vi "test_eet.vi"() -> ()   [LabVIEW 2023]
panel:
  out "lrv":sgl[](array[numeric])
  out "right_ray":sgl[](array[numeric])
  out "left_ray":sgl[](array[numeric])
  out "combined_ray":sgl[](array[numeric])
  out "valid":u32
  out "pose":sgl[][](array[numeric])
  in  "stop":bool
  in  "host":string="192.168.1.7"
  in  "path in":path=path "C:/Users/jcds/Documents/GitHub/hl2ss/extensions/client_labview/hl2ss_labview/hl2ss_ulm.dll"
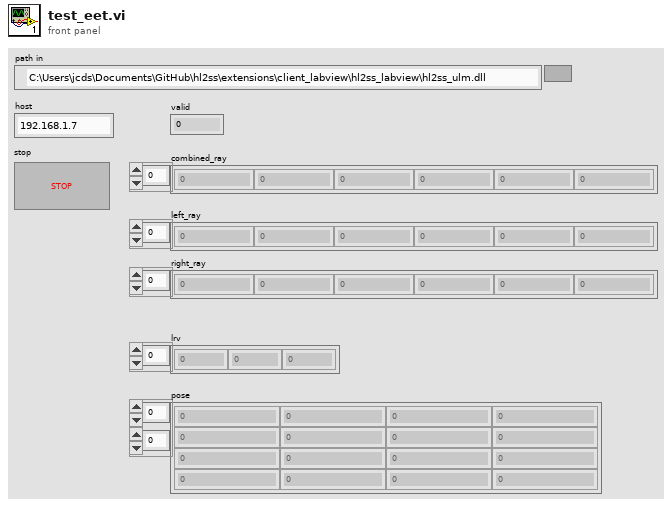
[diagram p1: front panel]
types:
  T1 = cluster{"chunk":u64, "framerate":u8, "_reserved_0":u8, "_reserved_1":u8, "_reserved_2":u8, "_reserved_3":u8, "_reserved_4":u8, "_reserved_5":u8, "_reserved_6":u8}
  T2 = cluster{"frame_stamp":i64, "timestamp":u64, "payload_size":u32, "status":i32, "payload":u64, "pose":u64}
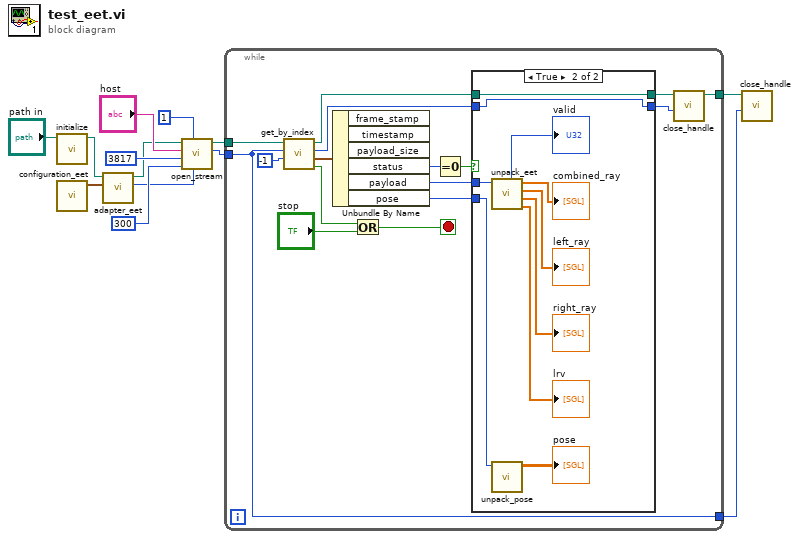
[diagram p0: block diagram]
diagram:
  n1 = call "initialize.vi"("path in"="path in") -> ("path out"=w4:path)  [unwired: 9 in, 1 out]
  n2 = call "configuration_eet.vi"() -> ("configuration_eet"=w5:T1)  [unwired: 11 in]
  n3 = call "adapter_eet.vi"("configuration_eet"=w5, "path in"=w4) -> ("configuration"=w2:u64, "path out"=w3:path)  [unwired: 8 in]
  n4 = call "open_stream.vi"("configuration"=w2, "decoded"=u8 1, "buffer_size"=u64 300, "port"=u16 3817, "host"="host", "path in"=w3) -> ("handle"=w9:u64, "path out"=w10:path)  [unwired: 3 in, 1 out]
  n5 = while {
    tunnel: w10 -> [w29]
    tunnel: w9 -> [w15]
    tunnel: [w16] -> w8
    tunnel: [w15] -> w7
    stop <- w27 stop-if-true
    n6 = call "get_by_index.vi"("frame_stamp"=i64 -1, "stream_handle"=w15, "path in"=w29) -> ("error"=w26:bool, "packet"=w24:T2, "packet_handle"=w19:u64, "path out"=w20:path)  [unwired: 5 in]
    n7 = Unbundle By Name(w24) -> ("status"=w22:i32, "payload"=w23:u64, "pose"=w14:u64)  [unwired: 3 out]
    n8 = Or(x=w26, y="stop") -> (x .or. y?=w27:bool)
    n9 = Equal To 0?(x=w22) -> (x = 0?=w21:bool)
    n10 = case shown="True" w21 {
      tunnel: w23 -> [_ w37]
      tunnel: w20 -> [w30 w41]
      tunnel: w19 -> [w31 w40]
      tunnel: [w30 w41] -> w18
      tunnel: [w31 w40] -> w17
      tunnel: w14 -> [_ w39]
      frame False {
      }
      frame True {
        n11 = call "unpack_eet.vi"("payload"=w37) -> ("lrv"=→"lrv":sgl[], "right_ray"=→"right_ray":sgl[], "left_ray"=→"left_ray":sgl[], "combined_ray"=→"combined_ray":sgl[], "valid"=→"valid":u32)  [unwired: 5 in, 1 out]
        n12 = call "unpack_pose.vi"("pose"=w39) -> ("pose"=→"pose":sgl[][])  [unwired: 9 in, 1 out]
      }
    }
    n13 = call "close_handle.vi"("handle"=w17, "path in"=w18) -> ("path out"=w16:path)  [unwired: 9 in]
  }
  n14 = call "close_handle.vi"("handle"=w7, "path in"=w8) -> ()  [unwired: 9 in, 1 out]
